vi "KEITHLEY-24XX-V-I.vi"() -> ()   [LabVIEW 2020]
uses:
  <instrlib>/Keithley 24XX/Public/Data/Read (Single Point).vi
  <instrlib>/Keithley 24XX/Keithley 24XX.lvlib
panel:
  in  "Compliance  Level (0.1)":dbl=0.1
  in  "Serial Configuration":T1={"Baud Rate"=9600, "Parity"=0, "Data Bits"=8, "Stop Bits"=10, "Flow Control"=0} {"Flow Control" items=["None", "XON/XOFF", "RTS/CTS", "XON/XOFF & RTS/CTS", "DTR/DSR", "XON/XOFF & DTR/DSR"]; "Stop Bits" items=["1.0"=10, "1.5"=15, "2.0"=20]; "Data Bits" items=["7"=7, "8"=8]; "Parity" items=["None", "Odd", "Even", "Mark", "Space"]; "Baud Rate" items=["300"=300, "600"=600, "1200"=1200, "2400"=2400, "4800"=4800, "9600"=9600, "19200"=19200]}
  in  "VISA resource name":refnum<visa-resource-name>
  out "Table Control":string[][](table)
  out "XY Graph 2":cluster{"ÇIKIÞ VOLTAJI":dbl[], "AKIM":dbl[]}(graph)
  in  "stop":bool
  out "GERÝLÝM":dbl[](array[numeric])
  in  "Step delay time":u32
  out "TERÝM SAYISI":dbl
  out "ÇIKIÞ AKIMI":dbl[](array[numeric])
  in  "Final current":dbl
  in  "Increment amount":dbl
  in  "Initial current":dbl
  in  "4W AYARI":bool=TRUE
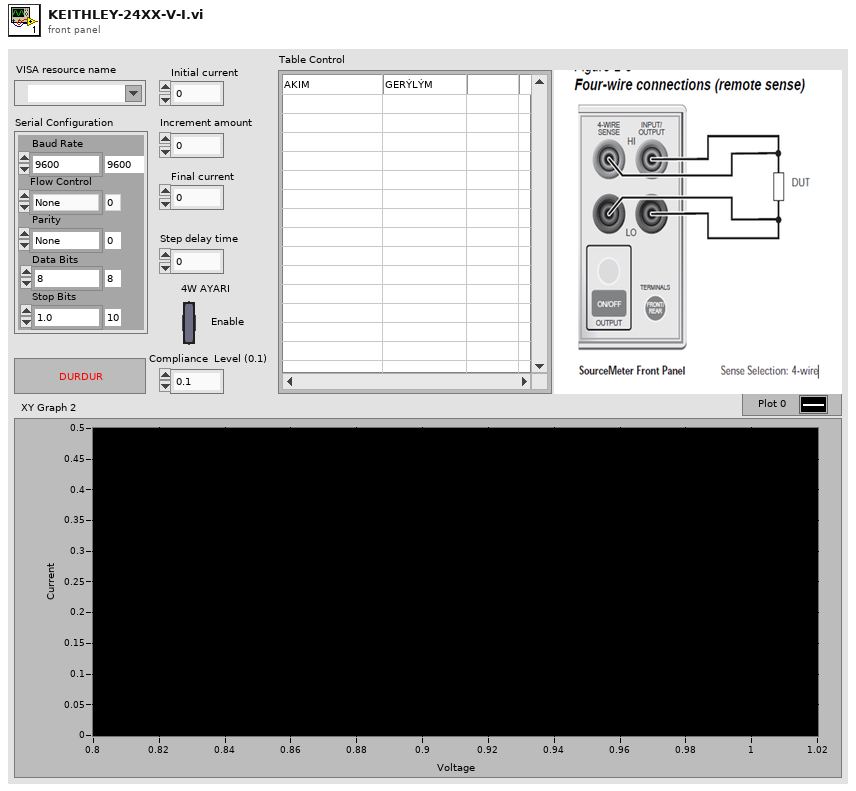
[diagram p1: front panel]
types:
  T1 = cluster{"Baud Rate":u32, "Parity":u16, "Data Bits":u16, "Stop Bits":u16, "Flow Control":u16}
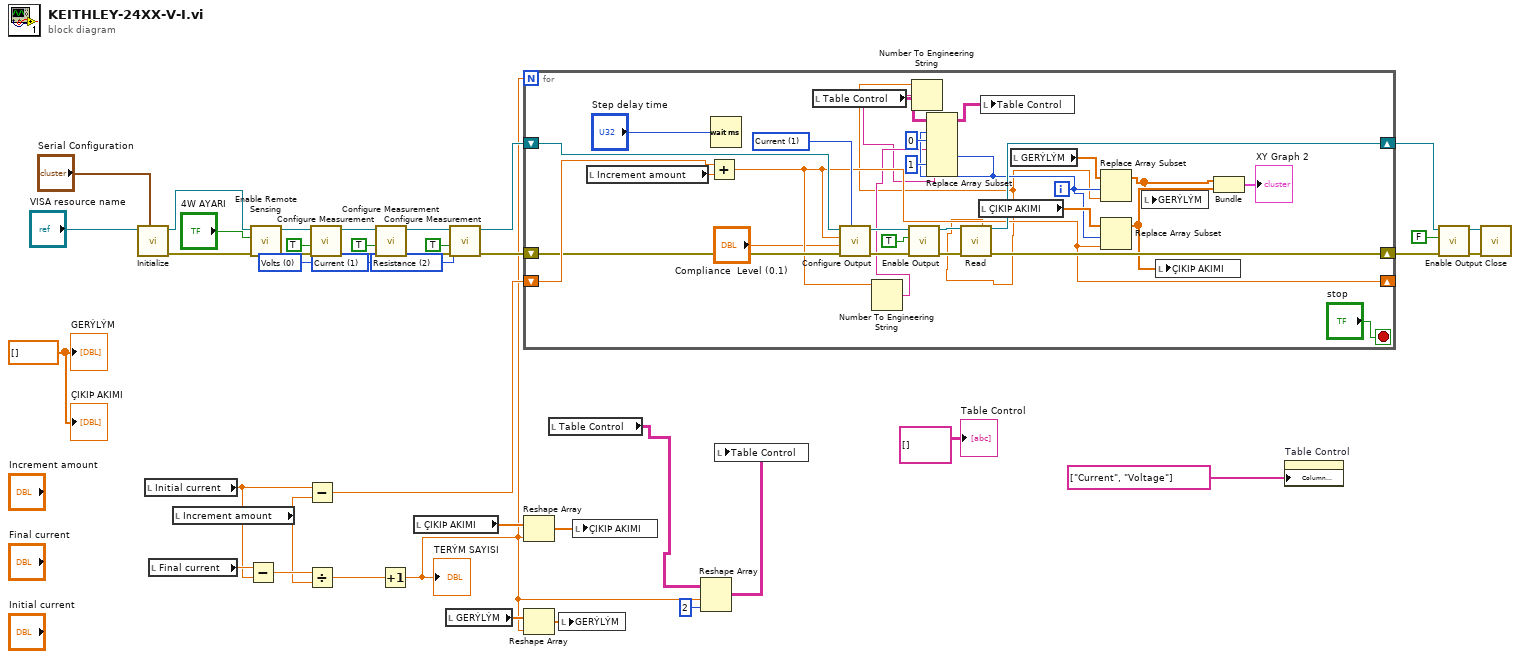
[diagram p0: block diagram]
diagram:
  w12 = u16 2 items=["Volts", "Current", "Resistance"] ("Function (0: Volts)")
  w13 = u16 1 items=["Volts", "Current", "Resistance"] ("Function (0: Volts)")
  w14 = u16 0 items=["Volts", "Current", "Resistance"] ("Function (0: Volts)")
  w17 = dbl[] []
  n1 = call <instrlib>:"Initialize.vi"("Serial Configuration"="Serial Configuration", "VISA resource name"="VISA resource name") -> ("error out"=w40:errorcluster, "VISA resource name out"=w41:refnum<visa-resource-name>)  [unwired: 8 in]
  n2 = local read "Initial current"() -> (w34:dbl)
  n3 = local read "Final current"() -> (w37:dbl)
  n4 = local read "Increment amount"() -> (w33:dbl)
  n5 = Subtract(x=w37, y=w34) -> (x-y=w36:dbl)
  n6 = call <instrlib>:"Enable Remote Sensing.vi"("error in (no error)"=w40, "Enable Remote Sensing (T: Enable)"="4W AYARI", "VISA resource name"=w41) -> ("error out"=w30:errorcluster, "VISA resource name out"=w31:refnum<visa-resource-name>)  [unwired: 7 in]
  n7 = Subtract(x=w34, y=w33) -> (x-y=w25:dbl)
  n8 = Divide(x=w36, y=w33) -> (x/y=w35:dbl)
  n9 = call <instrlib>:"Configure Measurement.vi"("error in (no error)"=w30, "Enable Auto Range (T:Enable)"=TRUE, "Function (0: Volts)"=w14, "VISA resource name"=w31) -> ("error out"=w28:errorcluster, "VISA resource name out"=w29:refnum<visa-resource-name>)  [unwired: 6 in]
  n10 = call <instrlib>:"Configure Measurement.vi"("error in (no error)"=w28, "Enable Auto Range (T:Enable)"=TRUE, "Function (0: Volts)"=w13, "VISA resource name"=w29) -> ("error out"=w26:errorcluster, "VISA resource name out"=w27:refnum<visa-resource-name>)  [unwired: 6 in]
  n11 = Increment(x=w35) -> (x+1=w5:dbl)
  "TERÝM SAYISI" <- w5
  n12 = local read "ÇIKIÞ AKIMI"() -> (w39:dbl[])
  n13 = local read "GERÝLÝM"() -> (w15:dbl[])
  n14 = call <instrlib>:"Configure Measurement.vi"("error in (no error)"=w26, "Enable Auto Range (T:Enable)"=TRUE, "Function (0: Volts)"=w12, "VISA resource name"=w27) -> ("error out"=w23:errorcluster, "VISA resource name out"=w24:refnum<visa-resource-name>)  [unwired: 6 in]
  n15 = for {
    N: w5 -> [_]
    shift-right: [w60] -> w18
    shift-left: w24 -> [w66]
    shift-right: [w59] -> w21
    shift-left: w23 -> [w65]
    shift-right: [w48] -> _
    shift-left: w25 -> [w68]
    i -> [w49]
    stop <- "stop" stop-if-true
    w57 = u16 1 items=["Voltage", "Current"] ("Source Mode  (0: Voltage)")
    n16 = local read "Increment amount"() -> (w70:dbl)
    n17 = Add(x=w68, y=w70) -> (x+y=w48:dbl)
    n18 = Wait (ms)(milliseconds to wait="Step delay time") -> ()  [unwired: 1 out]
    n19 = local read "Table Control"() -> (w53:string[][])
    n20 = call <instrlib>:"Configure Output.vi"("Source Mode  (0: Voltage)"=w57, "error in (no error)"=w65, "Compliance  Level (0.1)"="Compliance  Level (0.1)", "Output Level (0)"=w48, "VISA resource name"=w66) -> ("error out"=w63:errorcluster, "VISA resource name out"=w64:refnum<visa-resource-name>)  [unwired: 5 in]
    n21 = Number To Engineering String(4:w48) -> (0:w47:string)  [unwired: 3 in]
    n22 = call <instrlib>:"Enable Output.vi"("error in (no error)"=w63, "Enable Output (T: Enable)"=TRUE, "VISA resource name"=w64) -> ("error out"=w62:errorcluster, "VISA resource name out"=w61:refnum<visa-resource-name>)  [unwired: 7 in]
    n23 = call-poly <instrlib>:"Read.vi"("VISA resource name"=w61, "error in (no error)"=w62) -> ("Voltage"=w45:sgl, "VISA resource name out"=w60:refnum<visa-resource-name>, "error out"=w59:errorcluster)  [unwired: 7 in, 4 out]
    n24 = Number To Engineering String(4:w45) -> (0:w46:string)  [unwired: 3 in]
    n25 = Replace Array Subset(array=w53, new element #1=w47, index (row) #1=w49, index (col) #1=0 ("disabled index (col)"), new element #2=w46, index (row) #2=w49, index (col) #2=1 ("index (col)")) -> (w52:string[][])
    n26 = local read "ÇIKIÞ AKIMI"() -> (w69:dbl[])
    n27 = local write "Table Control"(w52) -> ()
    n28 = local read "GERÝLÝM"() -> (w56:dbl[])
    n29 = Replace Array Subset(array=w56, new element=w45, index=w49) -> (w42:dbl[])
    n30 = Replace Array Subset(array=w69, new element=w48, index=w49) -> (w43:dbl[])
    n31 = local write "GERÝLÝM"(w42) -> ()
    n32 = local write "ÇIKIÞ AKIMI"(w43) -> ()
    n33 = Bundle("GERÝLÝM"=w42, "ÇIKIÞ AKIMI"=w43) -> (→"XY Graph 2":cluster{"GERÝLÝM":dbl[], "ÇIKIÞ AKIMI":dbl[]})  [unwired: 1 in]
  }
  n34 = Reshape Array(w39, w5) -> (w38:dbl[])
  n35 = Reshape Array(w15, w5) -> (w16:dbl[])
  n36 = local read "Table Control"() -> (w7:string[][])
  n37 = local write "GERÝLÝM"(w16) -> ()
  n38 = local write "ÇIKIÞ AKIMI"(w38) -> ()
  n39 = Reshape Array(w7, w5, 2 ("dimension size")) -> (w6:string[][])
  n40 = local write "Table Control"(w6) -> ()
  n41 = property on="Table Control" class="Tbl (strict)"("Column Headers[]"=string[] ["Current", "Voltage"] ("Row Header Strings[]")) -> ()  [unwired: 2 in, 2 out]
  n42 = call <instrlib>:"Enable Output.vi"("error in (no error)"=w21, "Enable Output (T: Enable)"=FALSE, "VISA resource name"=w18) -> ("error out"=w20:errorcluster, "VISA resource name out"=w19:refnum<visa-resource-name>)  [unwired: 7 in]
  n43 = call <instrlib>:"Close.vi"("error in (no error)"=w20, "VISA resource name"=w19) -> ()  [unwired: 9 in, 1 out]
  "ÇIKIÞ AKIMI" <- w17
  "GERÝLÝM" <- w17
  "Table Control" <- string[][] [] ("Table Control")
